vi "Module Identities.vi"(8 "error in (no error)":errorcluster, 11 "Volatus Core in":refnum<class "Volatus Core.lvclass">) -> (0 "error out":errorcluster, 2 "Identities":refnum<class "Identity.lvclass">[](array[class]), 3 "Volatus Core out":refnum<class "Volatus Core.lvclass">)   [LabVIEW 2020, in "Volatus.lvlib" / "Volatus Core.lvclass"]
uses:
  Volatus Core.lvclass
  Identity/Identity.lvclass
  Volatus Core Identity/Volatus Core Identity.lvclass
  C:/dev/lv20CE/relink/lv-volatus/Volatus/Identity/Identity.lvclass
  Volatus Core.lvclass/Volatus Core.ctl
  Status Tree Identity/Status Tree Identity.lvclass
  C:/dev/lv20CE/relink/lv-volatus/Volatus/Volatus Core Identity/Volatus Core Identity.lvclass
  C:/dev/lv20CE/relink/lv-volatus/Volatus/Status Tree Identity/Status Tree Identity.lvclass
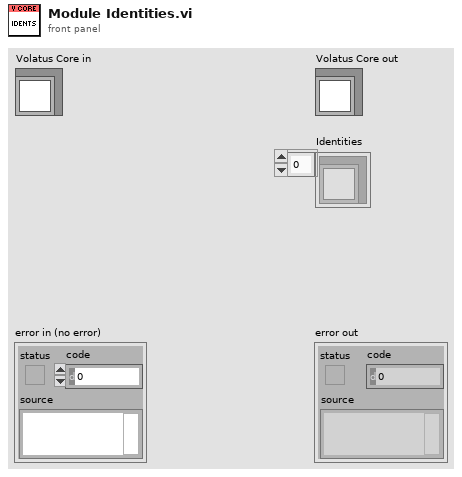
[diagram p1: front panel]
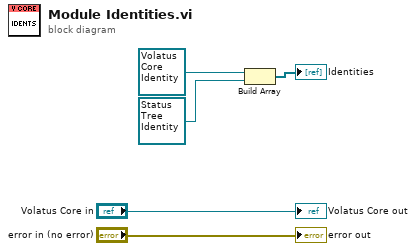
[diagram p0: block diagram]
diagram:
  n1 = Build Array(refnum<class "Volatus Core Identity.lvclass"> refnum ("Volatus:Volatus Core Identity.lvclass"), refnum<class "Status Tree Identity.lvclass"> refnum ("Volatus:Status Tree Identity.lvclass")) -> (→"Identities":refnum<class "Identity.lvclass">[])
  "error out" <- "error in (no error)"
  "Volatus Core out" <- "Volatus Core in"
